vi "手动启动选择对话框.vi"() -> (2 "确定":bool, 3 "输出簇":T1)   [LabVIEW 2016, in "PLC.lvlib"]
uses:
  PLC.lvlib
panel:
  in  "自动运行启动参数":T2
  in  "测试模式":enum16{"正常测试", "集成干预"}(ring)
  in  "取消":bool
  in  "确定":bool
  # "请选择启动参数"
  # "请选择启动模式："
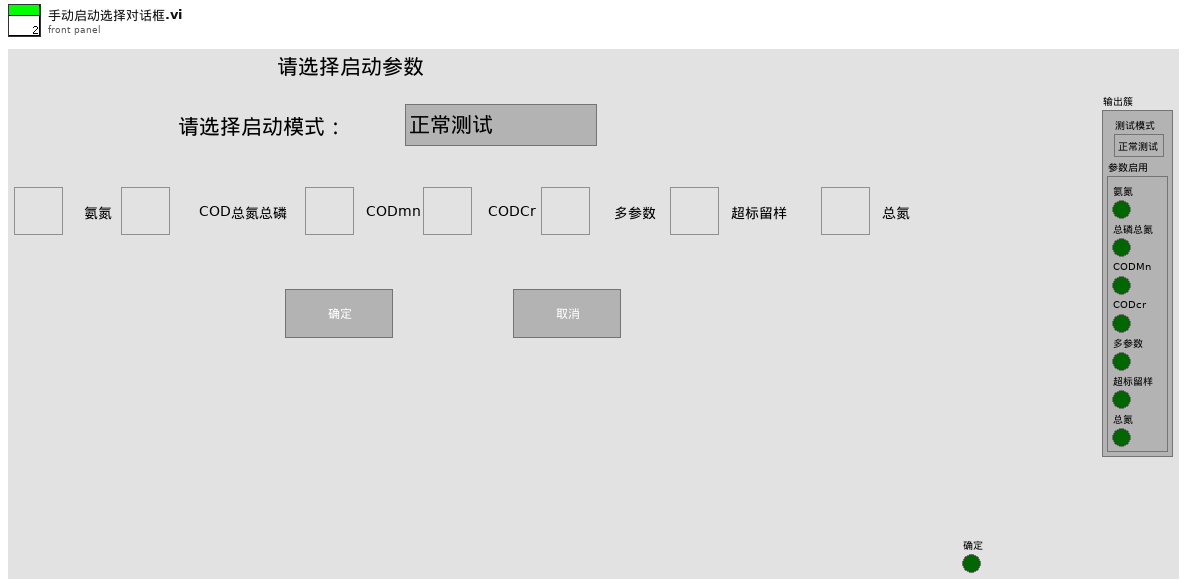
[diagram p1: front panel]
types:
  T1 = cluster{"测试模式":enum16{"正常测试", "集成干预"}, "参数启用":cluster{"氨氮":bool, "总磷总氮":bool, "CODMn":bool, "CODcr":bool, "多参数":bool, "超标留样":bool, "总氮":bool}}
  T2 = cluster{"氨氮":bool, "总磷总氮":bool, "CODmn":bool, "CODCr":bool, "多参数":bool, "超标留样":bool, "总氮":bool}
  T3 = cluster{"COD":bool, "氨氮":bool, "总氮":bool, "总磷":bool}
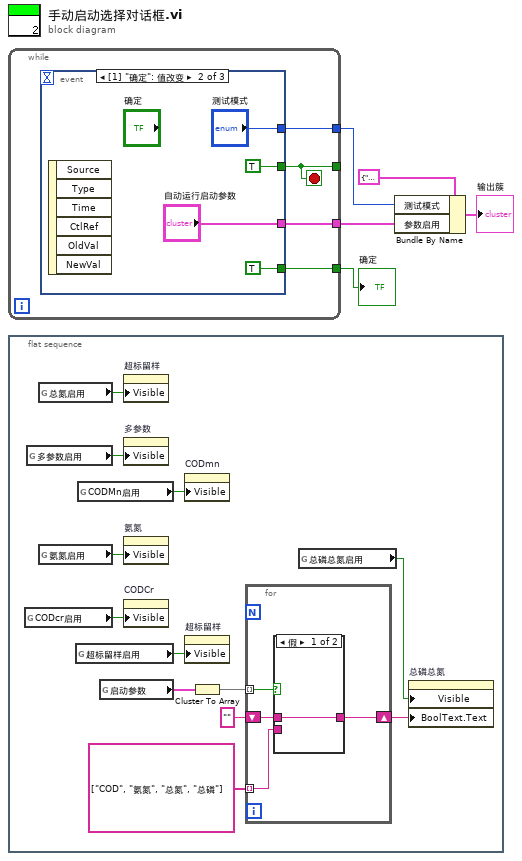
[diagram p0: block diagram]
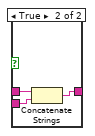
[diagram p2: hidden frame]
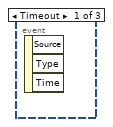
[diagram p3: hidden frame]
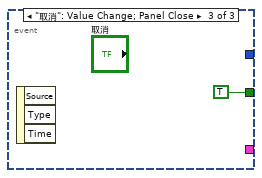
[diagram p4: hidden frame]
diagram:
  n1 = while {
    tunnel: [w9] -> w1
    tunnel: [w8] -> _
    tunnel: [w7] -> w5
    tunnel: [w6] -> w4
    stop <- w8 stop-if-true
    n2 = event shown="[1] \"确定\": 值改变" {
      selector: _ -> [_ _ _]
      dyn-events: _ -> [_ _ _]
      timeout: _ -> [_ _ _]
      tunnel: [_ TRUE TRUE] -> w8
      tunnel: [_ "自动运行启动参数" _] -> w9
      tunnel: [_ TRUE _] -> w7
      tunnel: [_ "测试模式" _] -> w6
      event Timeout {
        n3 = event-data() -> ()  [unwired: 1 in, 3 out]
      }
      event "确定": Value Change {
        n4 = event-data() -> ()  [unwired: 1 in, 6 out]
      }
      event "取消": Value Change; Panel Close {
        n5 = event-data() -> ()  [unwired: 1 in, 3 out]
      }
    }
  }
  "确定" <- w5
  n6 = flat-sequence {
    frame #0 {
      n7 = global read "系统设置全局变量.vi" "CODcr启用"() -> (w26:bool)
      n8 = global read "系统设置全局变量.vi" "多参数启用"() -> (w23:bool)
      n9 = global read "系统设置全局变量.vi" "总氮启用"() -> (w20:bool)
      n10 = global read "系统设置全局变量.vi" "氨氮启用"() -> (w24:bool)
      n11 = global read "系统设置全局变量.vi" "超标留样启用"() -> (w21:bool)
      n12 = global read "系统设置全局变量.vi" "CODMn启用"() -> (w25:bool)
      n13 = global read "总磷总氮断电保存全局变量.vi" "启动参数"() -> (w18:T3)
      n14 = property on="超标留样" class="Bool (严格)"("Visible"=w20) -> ()  [unwired: 2 in, 2 out]
      n15 = property on="多参数" class="Bool (严格)"("Visible"=w23) -> ()  [unwired: 2 in, 2 out]
      n16 = property on="氨氮" class="Bool (严格)"("Visible"=w24) -> ()  [unwired: 2 in, 2 out]
      n17 = property on="CODCr" class="Bool (严格)"("Visible"=w26) -> ()  [unwired: 2 in, 2 out]
      n18 = property on="CODmn" class="Bool (严格)"("Visible"=w25) -> ()  [unwired: 2 in, 2 out]
      n19 = property on="超标留样" class="Bool (严格)"("Visible"=w21) -> ()  [unwired: 2 in, 2 out]
      n20 = Cluster To Array(cluster=w18) -> (array=w19:bool[])
      n21 = for {
        tunnel: string[] ["COD", "氨氮", "总氮", "总磷"] -> [w30] mode=indexing
        shift-right: [w29] -> w15
        shift-left: "" -> [w28]
        tunnel: w19 -> [w27] mode=indexing
        n22 = case shown="假" w27 {
          tunnel: w30 -> [_ w34]
          tunnel: [w31 w33] -> w29
          tunnel: w28 -> [w31 w32]
          frame False {
          }
          frame True {
            n23 = Concatenate Strings(w32, w34) -> (w33:string)
          }
        }
      }
      n24 = global read "系统设置全局变量.vi" "总磷总氮启用"() -> (w22:bool)
      n25 = property on="总磷总氮" class="Bool (严格)"("Visible"=w22, "BoolText.Text"=w15) -> ()  [unwired: 2 in, 2 out]
    }
  }
  n26 = Bundle By Name(cluster=T1 {"测试模式"=enum."正常测试", "参数启用"={"氨氮"=FALSE, "总磷总氮"=FALSE, "CODMn"=FALSE, "CODcr"=FALSE, "多参数"=FALSE, "超标留样"=FALSE, "总氮"=FALSE}} ("参数"), "测试模式"=w4, "参数启用"=w1) -> (→"输出簇":T1)
